vi "TestSVGParse.vi"(8 "error in (no error)":errorcluster) -> (0 "error out":errorcluster)   [LabVIEW 2019]
uses:
  ParseXML/Rect.ctl
  ParseXML/Path.ctl
  ParseXML/ParseSVG.lvclass
  ParseXML/Image.ctl
  ParseXML/ParseSVG.lvclass/ParseSVG.ctl
  <vilib>/addons/_JKI Toolkits/Caraya/classes/Assert/Assert Equal Value and Type_Variant.vi
  <vilib>/addons/_JKI Toolkits/Caraya/classes/Assert/Assert Equal Value_Variant.vi
  <vilib>/addons/_JKI Toolkits/Caraya/classes/Test/Test.lvclass
  <vilib>/addons/_JKI Toolkits/Caraya/classes/Assert/Assert.lvclass
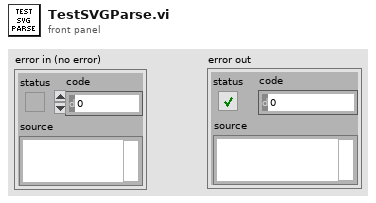
[diagram p1: front panel]
types:
  T1 = typedef "ParseSVG.lvclass/Image.ctl" = cluster{"x":string, "y":string, "width":string, "height":string, "xlink:href":string, "id":string}
  T2 = typedef "ParseSVG.lvclass/Path.ctl" = cluster{"d":string, "style":string, "transform":string, "id":string}
  T3 = typedef "ParseSVG.lvclass/Rect.ctl" = cluster{"style":string, "transform":string, "x":string, "y":string, "width":string, "height":string, "rx":string, "ry":string, "id":string}
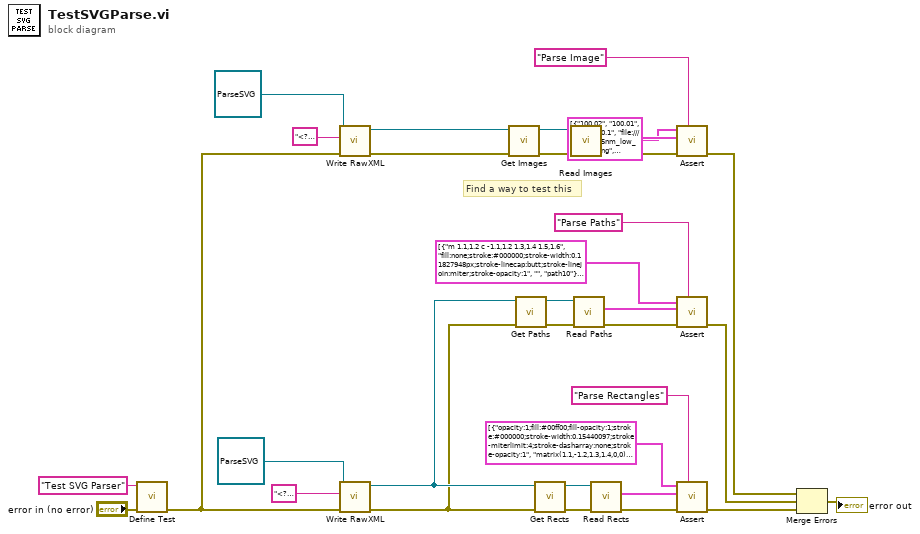
[diagram p0: block diagram]
diagram:
  # "Find a way to test this"
  n1 = call <vilib>:"Define Test.vi"("error in (no error)"="error in (no error)", "Label (VI Title)"="Test SVG Parser") -> ("error out"=w1:errorcluster)  [unwired: 8 in, 1 out]
  n2 = call "Write RawXML.vi"("error in (no error)"=w1, "RawXML"="<?xml version=\"1.0\" encoding=\"UTF-8\" standalone=\"no\"?>\n<!-- Created with Inkscape (http://www.inkscape.org/) -->\n\n<svg\n   xmlns:dc=\"http://purl.org/dc/elements/1.1/\"\n   xmlns:cc=\"http://creativecommons.org/ns#\"\n   xmlns:rdf=\"http://www.w3.org/1999/02/22-rdf-syntax-ns#\"\n   xmlns:svg=\"http://www.w3.org/2000/svg\"\n   xmlns=\"http://www.w3.org/2000/svg\"\n   xmlns:xlink=\"http://www.w3.org/1999/xlink\"\n   xmlns:sodipodi=\"http://sodipodi.sourceforge.net/DTD/sodipodi-0.dtd\"\n   xmlns:inkscape=\"http://www.inkscape.org/namespaces/inkscape\"\n   width=\"210mm\"\n   height=\"297mm\"\n   viewBox=\"0 0 210 297\"\n   version=\"1.1\"\n   id=\"svg8\"\n   inkscape:version=\"0.92.4 (5da689c313, 2019-01-14)\"\n   sodipodi:docname=\"Rotated Rectangle.svg\">\n  <defs\n     id=\"defs2\" />\n  <sodipodi:namedview\n     id=\"base\"\n     pagecolor=\"#ffffff\"\n     bordercolor=\"#666666\"\n     borderopacity=\"1.0\"\n     inkscape:pageopacity=\"0.0\"\n     inkscape:pageshadow=\"2\"\n     inkscape:zoom=\"1.979899\"\n     inkscape:cx=\"490.72081\"\n     inkscape:cy=\"632.73714\"\n     inkscape:document-units=\"mm\"\n     inkscape:current-layer=\"layer1\"\n     showgrid=\"false\"\n     inkscape:window-width=\"1920\"\n     inkscape:window-height=\"1001\"\n     inkscape:window-x=\"-9\"\n     inkscape:window-y=\"-9\"\n     inkscape:window-maximized=\"1\" />\n  <metadata\n     id=\"metadata5\">\n    <rdf:RDF>\n      <cc:Work\n         rdf:about=\"\">\n        <dc:format>image/svg+xml</dc:format>\n        <dc:type\n           rdf:resource=\"http://purl.org/dc/dcmitype/StillImage\" />\n        <dc:title></dc:title>\n      </cc:Work>\n    </rdf:RDF>\n  </metadata>\n  <g\n     inkscape:label=\"Layer 1\"\n     inkscape:groupmode=\"layer\"\n     id=\"layer1\">\n    <rect\n       style=\"opacity:1;fill:#00ff00;fill-opacity:1;stroke:#000000;stroke-width:0.2;stroke-miterlimit:4;stroke-dasharray:none;stroke-opacity:1\"\n       id=\"rect10\"\n       width=\"91.470238\"\n       height=\"73.327377\"\n       x=\"-154.84225\"\n       y=\"86.601273\"\n       transform=\"rotate(-75.111271)\" />\n    <rect\n       style=\"opacity:1;fill:#00ff00;fill-opacity:1;stroke:#000000;stroke-width:0.2;stroke-miterlimit:4;stroke-dasharray:none;stroke-opacity:1\"\n       id=\"rect12\"\n       width=\"76.351196\"\n       height=\"58.964287\"\n       x=\"-120.4144\"\n       y=\"98.469505\"\n       inkscape:transform-center-x=\"33.251622\"\n       inkscape:transform-center-y=\"66.085109\"\n       transform=\"rotate(-74.485231)\" />\n    <image\n       sodipodi:absref=\"C:\\gold_75nm_low_voltage.png\"\n       y=\"100.01\"\n       x=\"100.02\"\n       id=\"image33\"\n       xlink:href=\"file:///C:/gold_75nm_low_voltage.png\"\n       preserveAspectRatio=\"none\"\n       height=\"70.1\"\n       width=\"50.3\" />\n  </g>\n</svg>", "ParseSVG.lvclass"=refnum<class "ParseSVG.lvclass"> refnum ("ParseXML in")) -> ("error out"=w12:errorcluster, "ParseSVG.lvclass 2"=w13:refnum<class "ParseSVG.lvclass">)  [unwired: 7 in]
  n3 = call "Write RawXML.vi"("error in (no error)"=w1, "RawXML"="<?xml version=\"1.0\" encoding=\"UTF-8\" standalone=\"no\"?>\n<!-- Created with Inkscape (http://www.inkscape.org/) -->\n\n<svg\n   xmlns:dc=\"http://purl.org/dc/elements/1.1/\"\n   xmlns:cc=\"http://creativecommons.org/ns#\"\n   xmlns:rdf=\"http://www.w3.org/1999/02/22-rdf-syntax-ns#\"\n   xmlns:svg=\"http://www.w3.org/2000/svg\"\n   xmlns=\"http://www.w3.org/2000/svg\"\n   xmlns:sodipodi=\"http://sodipodi.sourceforge.net/DTD/sodipodi-0.dtd\"\n   xmlns:inkscape=\"http://www.inkscape.org/namespaces/inkscape\"\n   width=\"210mm\"\n   height=\"297mm\"\n   viewBox=\"0 0 210 297\"\n   version=\"1.1\"\n   id=\"svg8\"\n   inkscape:version=\"0.92.4 (5da689c313, 2019-01-14)\"\n   sodipodi:docname=\"TestDrawing.svg\">\n  <defs\n     id=\"defs2\" />\n  <sodipodi:namedview\n     id=\"base\"\n     pagecolor=\"#ffffff\"\n     bordercolor=\"#666666\"\n     borderopacity=\"1.0\"\n     inkscape:pageopacity=\"0.0\"\n     inkscape:pageshadow=\"2\"\n     inkscape:zoom=\"0.35\"\n     inkscape:cx=\"-614.28572\"\n     inkscape:cy=\"560\"\n     inkscape:document-units=\"mm\"\n     inkscape:current-layer=\"layer1\"\n     showgrid=\"false\"\n     inkscape:window-width=\"1920\"\n     inkscape:window-height=\"1001\"\n     inkscape:window-x=\"-9\"\n     inkscape:window-y=\"-9\"\n     inkscape:window-maximized=\"1\" />\n  <metadata\n     id=\"metadata5\">\n    <rdf:RDF>\n      <cc:Work\n         rdf:about=\"\">\n        <dc:format>image/svg+xml</dc:format>\n        <dc:type\n           rdf:resource=\"http://purl.org/dc/dcmitype/StillImage\" />\n        <dc:title />\n      </cc:Work>\n    </rdf:RDF>\n  </metadata>\n  <g\n     inkscape:label=\"Layer 1\"\n     inkscape:groupmode=\"layer\"\n     id=\"layer1\">\n    <path\n       style=\"fill:none;stroke:#000000;stroke-width:0.11827948px;stroke-linecap:butt;stroke-linejoin:miter;stroke-opacity:1\"\n       d=\"m 1.1,1.2 c -1.1,1.2 1.3,1.4 1.5,1.6\"\n       id=\"path10\"\n       inkscape:connector-curvature=\"0\" />\n    <path\n       style=\"fill:none;stroke:#000000;stroke-width:0.26458332px;stroke-linecap:butt;stroke-linejoin:miter;stroke-opacity:100\"\n       d=\"M 10.1,10.2 10.3,10.4\"\n       id=\"path12\"\n       inkscape:connector-curvature=\"0\" />\n    <rect\n       style=\"opacity:1;fill:#00ff00;fill-opacity:1;stroke:#000000;stroke-width:0.15440097;stroke-miterlimit:4;stroke-dasharray:none;stroke-opacity:1\"\n       id=\"rect9\"\n       width=\"1.1\"\n       height=\"1.2\"\n       x=\"-1.1\"\n       y=\"-1.2\"\n       transform=\"matrix(1.1,-1.2,1.3,1.4,0,0)\" />\n    <rect\n       style=\"opacity:100;fill:#00ff00;fill-opacity:1;stroke:#000000;stroke-width:0.15440097;stroke-miterlimit:4;stroke-dasharray:none;stroke-opacity:1\"\n       id=\"rect9\"\n       width=\"10.1\"\n       height=\"10.2\"\n       x=\"-10.1\"\n       y=\"-10.2\"\n       transform=\"matrix(10.1,-10.2,10.3,10.4,0,0)\" />\n  </g>\n</svg>", "ParseSVG.lvclass"=refnum<class "ParseSVG.lvclass"> refnum ("ParseXML in")) -> ("error out"=w3:errorcluster, "ParseSVG.lvclass 2"=w14:refnum<class "ParseSVG.lvclass">)  [unwired: 7 in]
  n4 = call "Get Images.vi"("error in (no error)"=w12, "ParseSVG in"=w13) -> ("error out"=w8:errorcluster, "ParseSVG out"=w11:refnum<class "ParseSVG.lvclass">)  [unwired: 8 in]
  n5 = call "Get Paths.vi"("error in (no error)"=w3, "ParseXML in"=w14) -> ("error out"=w25:errorcluster, "ParseXML out"=w26:refnum<class "ParseSVG.lvclass">)  [unwired: 8 in]
  n6 = call "Get Rects.vi"("error in (no error)"=w3, "ParseSVG in"=w14) -> ("error out"=w29:errorcluster, "ParseSVG out"=w33:refnum<class "ParseSVG.lvclass">)  [unwired: 8 in]
  n7 = call "Read Images.vi"("error in (no error)"=w8, "ParseSVG in"=w11) -> ("error out"=w2:errorcluster, "Images"=w7:T1[])  [unwired: 7 in, 1 out]
  n8 = call "Read Paths.vi"("error in (no error)"=w25, "ParseXML in"=w26) -> ("error out"=w24:errorcluster, "Paths"=w23:T2[])  [unwired: 7 in, 1 out]
  n9 = call "Read Rects.vi"("error in (no error)"=w29, "ParseSVG in"=w33) -> ("error out"=w28:errorcluster, "Rects"=w31:T3[])  [unwired: 7 in, 1 out]
  n10 = call-poly <vilib>:"Assert.vi"("Label"="Parse Image", "error in (no error)"=w2, "Y"=w7, "X"=T1[] [{"x"="100.02", "y"="100.01", "width"="50.3", "height"="70.1", "xlink:href"="file:///C:/gold_75nm_low_voltage.png", "id"="image33"}] ("Images")) -> ("error out"=w4:errorcluster)  [unwired: 6 in, 1 out]
  n11 = call-poly <vilib>:"Assert.vi"("Label"="Parse Paths", "error in (no error)"=w24, "Y"=w23, "X"=T2[] [{"d"="m 1.1,1.2 c -1.1,1.2 1.3,1.4 1.5,1.6", "style"="fill:none;stroke:#000000;stroke-width:0.11827948px;stroke-linecap:butt;stroke-linejoin:miter;stroke-opacity:1", "transform"="", "id"="path10"}, {"d"="M 10.1,10.2 10.3,10.4", "style"="fill:none;stroke:#000000;stroke-width:0.26458332px;stroke-linecap:butt;stroke-linejoin:miter;stroke-opacity:100", "transform"="", "id"="path12"}] ("Paths")) -> ("error out"=w20:errorcluster)  [unwired: 6 in, 1 out]
  n12 = call-poly <vilib>:"Assert.vi"("Label"="Parse Rectangles", "error in (no error)"=w28, "Y"=w31, "X"=T3[] [{"style"="opacity:1;fill:#00ff00;fill-opacity:1;stroke:#000000;stroke-width:0.15440097;stroke-miterlimit:4;stroke-dasharray:none;stroke-opacity:1", "transform"="matrix(1.1,-1.2,1.3,1.4,0,0)", "x"="-1.1", "y"="-1.2", "width"="1.1", "height"="1.2", "rx"="", "ry"="", "id"="rect9"}, {"style"="opacity:100;fill:#00ff00;fill-opacity:1;stroke:#000000;stroke-width:0.15440097;stroke-miterlimit:4;stroke-dasharray:none;stroke-opacity:1", "transform"="matrix(10.1,-10.2,10.3,10.4,0,0)", "x"="-10.1", "y"="-10.2", "width"="10.1", "height"="10.2", "rx"="", "ry"="", "id"="rect9"}] ("Rects")) -> ("error out"=w19:errorcluster)  [unwired: 6 in, 1 out]
  n13 = Merge Errors(w4, w20, w19) -> (→"error out":errorcluster)
